vi "get InteractionParameterReceived element by name.vi"(10 "name":string, 11 "interaction_attribute_type":T1) -> (1 "found":bool, 3 "element out":dbl)   [LabVIEW 2019, in "HLA Custom Device Engine.lvlib"]
uses:
  HLA Custom Device Engine.lvlib
  emea-ni-adg-hla-lv/src/library/typedefs/OrderType.ctl
  emea-ni-adg-hla-lv/src/library/openrti_rti1516eLv.lvlib
  emea-ni-adg-hla-lv/src/library/typedefs/TransportationType.ctl
  interaction_info_received_type.ctl
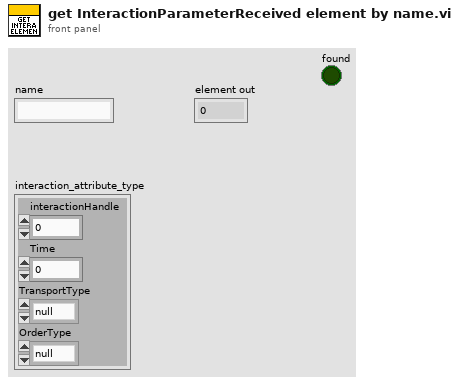
[diagram p1: front panel]
types:
  T1 = typedef "HLA Custom Device Engine.lvlib/interaction_info_received_type.ctl" = cluster{"interactionHandle":u64, "Time":u32, "TransportType":T2, "OrderType":T3}
  T2 = typedef "openrti_rti1516eLv.lvlib/TransportationType.ctl" = enum32{"null", "RELIABLE", "BEST_EFFORT"}
  T3 = typedef "openrti_rti1516eLv.lvlib/OrderType.ctl" = enum32{"null", "RECEIVE", "TIMESTAMP"}
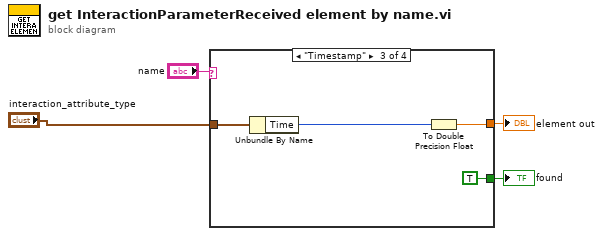
[diagram p0: block diagram]
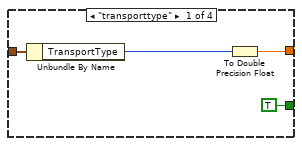
[diagram p2: hidden frame]
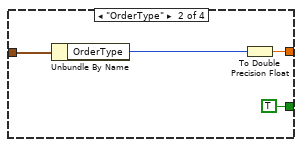
[diagram p3: hidden frame]
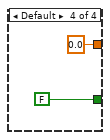
[diagram p4: hidden frame]
diagram:
  n1 = case shown="\"Timestamp\"" "name" {
    tunnel: "interaction_attribute_type" -> [w7 w12 w15 _]
    tunnel: [w6 w11 w14 0.0] -> w2
    tunnel: [TRUE TRUE TRUE FALSE] -> w1
    frame "transporttype" {
      n2 = Unbundle By Name(w7) -> ("TransportType"=w8:T2)
      n3 = To Double Precision Float(number=w8) -> (double precision float=w6:dbl)
    }
    frame "OrderType" {
      n4 = Unbundle By Name(w12) -> ("OrderType"=w10:T3)
      n5 = To Double Precision Float(number=w10) -> (double precision float=w11:dbl)
    }
    frame "Timestamp" {
      n6 = Unbundle By Name(w15) -> ("Time"=w16:u32)
      n7 = To Double Precision Float(number=w16) -> (double precision float=w14:dbl)
    }
    frame Default {
    }
  }
  "element out" <- w2
  "found" <- w1
